vi "Play.vi"(8 "error in (no error)":errorcluster, 11 "Player in":refnum<class "Player.lvclass">) -> (0 "error out":errorcluster, 3 "Player out":refnum<class "Player.lvclass">)   [LabVIEW 2016, in "Player.lvclass"]
uses:
  Player.lvclass
  Dice/Dice.lvclass
  Dice/Dice.lvclass/Dice.ctl
  Player.lvclass/Player.ctl
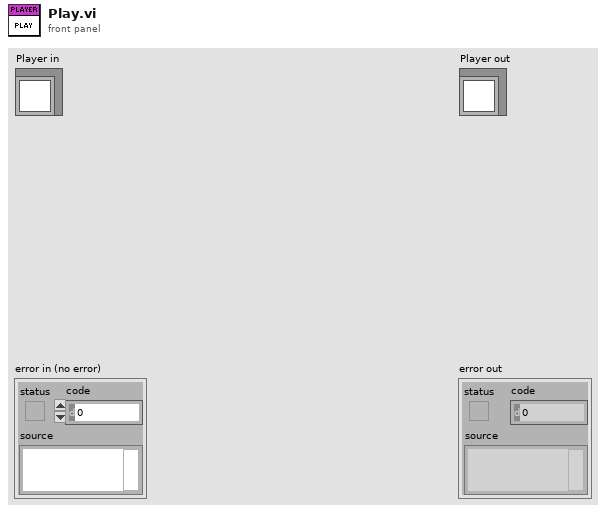
[diagram p1: front panel]
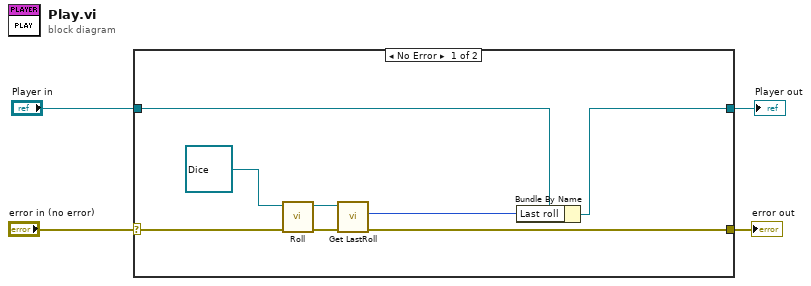
[diagram p0: block diagram]
diagram:
  n1 = case shown="No Error" "error in (no error)" {
    selector: "error in (no error)" -> [w10 w14]
    tunnel: [w6 w14] -> w3
    tunnel: [w5 w13] -> w1
    tunnel: "Player in" -> [w8 w13]
    frame No Error {
      n2 = call "Roll.vi"("error in (no error)"=w10, "Dice in"=refnum<class "Dice.lvclass"> refnum ("Dice.lvclass")) -> ("error out"=w11:errorcluster, "Dice out"=w12:refnum<class "Dice.lvclass">)  [unwired: 8 in]
      n3 = call "Get LastRoll.vi"("error in (no error)"=w11, "Dice in"=w12) -> ("error out"=w6:errorcluster, "LastRoll"=w7:u8)  [unwired: 7 in, 1 out]
      n4 = Bundle By Name(cluster=w8, "Last roll"=w7) -> (w5:refnum<class "Player.lvclass">)
    }
    frame Error {
    }
  }
  "error out" <- w3
  "Player out" <- w1
